vi "XML Script - Append Terminal Name (Shift Register -  Left).vi"(1 "shiftreg":string) -> (0 "shiftreg.Left":string)   [LabVIEW 2020]
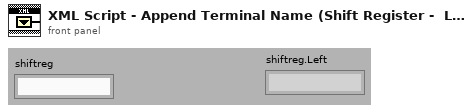
[diagram p1: front panel]
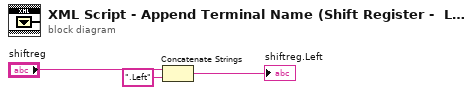
[diagram p0: block diagram]
diagram:
  n1 = Concatenate Strings("shiftreg", ".Left" ("string")) -> (→"shiftreg.Left":string)
